vi "Get Old Tweets - Finite.vi"() -> ()   [LabVIEW 2011]
doc: "This example gets a finite number of old tweets starting the top of the user's timeline. This example behaves the same way as Get New Tweets- Finte if the Twitter Handle is not saved to a shift register."
uses:
  Controls/Tweet.ctl
  i3-twitter.lvlib
panel:
  out "Tweets Read":T1[](array[typedef])
  out "Time Stamp of Oldest Tweet":timestamp
  in  "Screen Name (Empty)":string
  out "Num of Tweets Read":i32
  in  "Num of Tweets to Read":i32
  in  "Consumer Key":string
  in  "Consumer Secret":string
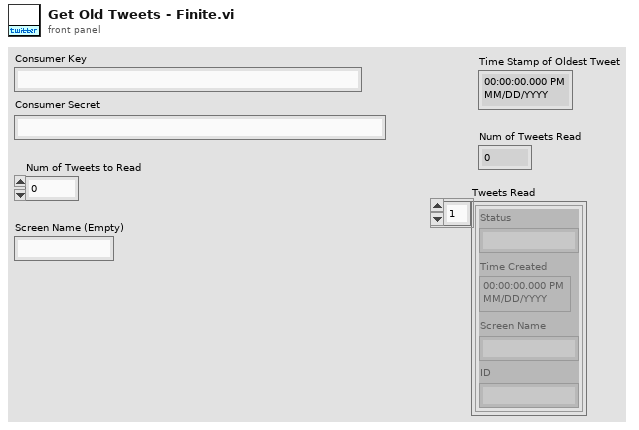
[diagram p1: front panel]
types:
  T1 = typedef "i3-twitter.lvlib/Tweet.ctl" = cluster{"Status":string, "Time Created":timestamp, "Screen Name":string, "ID":string}
  T2 = typedef "i3-twitter.lvlib/Twitter Handle.ctl" = cluster{"OAuth Credentials":T3, "since ID":string, "max ID":string, "Screen Name":string}
  T3 = typedef "i3-oauth.lvlib/OAuth Credentials.ctl" = cluster{"Consumer Key":string, "Signature Method":T4, "Token":string, "Version":string, "Token Secret":string, "Consumer Secret":string}
  T4 = typedef "i3-oauth.lvlib/Signature Method.ctl" = enum16{"HMAC-MD5", "HMAC-SHA1", "HMAC-SHA224", "HMAC-SHA256", "HMAC-SHA384", "HMAC-SHA512"}
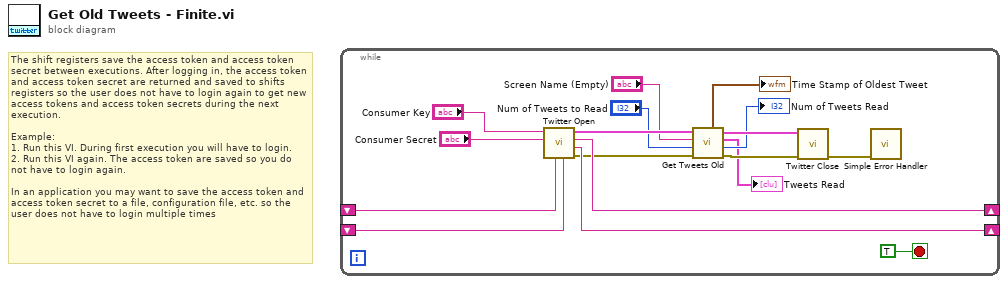
[diagram p0: block diagram]
diagram:
  # "The shift registers save the access token and access token secret between executions. After logging in, the access token and access token secret are returned and saved to shifts registers so the user does not have to login again to get new access tokens and access token secrets during the next execution.\n\nExample:\n1. Run this VI. During first execution you will have to login.\n2. Run this VI again. The access token are saved so you do not have to login again.\n\nIn an application you may want to save the access token and access token secret to a file, configuration file, etc. so the user does not have to login multiple times"
  n1 = while {
    shift-right: [w12] -> _
    shift-left: _ -> [w2]
    shift-right: [w11] -> _
    shift-left: _ -> [w1]
    stop <- TRUE stop-if-true
    n2 = call "Twitter Open.vi"("Access Token Secret (In)"=w1, "Access Token (In)"=w2, "Consumer Secret"="Consumer Secret", "Consumer Key"="Consumer Key") -> ("error out"=w10:errorcluster, "Access Token Secret (Out)"=w11:string, "Access Token (Out)"=w12:string, "Twitter Handle Out"=w15:T2)  [unwired: 4 in]
    n3 = call "Get Tweets Old.vi"("error in"=w10, "Tweets to Read (10)"="Num of Tweets to Read", "Screen Name (Empty)"="Screen Name (Empty)", "Twitter Handle In"=w15) -> ("error out"=w14:errorcluster, "Actual Num of Tweets Read"=→"Num of Tweets Read":i32, "Old Tweets Read"=→"Tweets Read":T1[], "Twitter Handle Out"=w13:T2, "Time Stamp of Oldest Tweet"=→"Time Stamp of Oldest Tweet":timestamp)  [unwired: 3 in]
    n4 = call "Twitter Close.vi"("error in"=w14, "Twitter Handle In"=w13) -> ("error in"=w8:errorcluster)  [unwired: 9 in]
    n5 = call <vilib>:"Simple Error Handler.vi"("error in (no error)"=w8) -> ()  [unwired: 4 in, 5 out]
  }
